vi "copy node from reference.vi"(8 "error in":errorcluster, 11 "TBM node dvr":refnum<data-value>) -> (0 "error out":errorcluster, 3 "TBM node value":refnum<class "TBM Configuration Node.lvclass">)   [LabVIEW 2013, in "PL Framework Configuration Tool.lvlib" / "TBM Configuration Node.lvclass"]
uses:
  TBM Configuration Node.lvclass
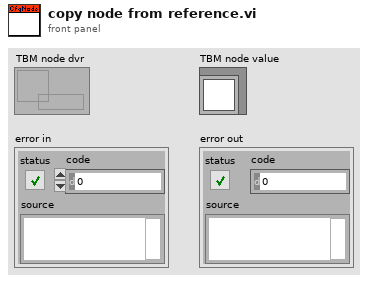
[diagram p1: front panel]
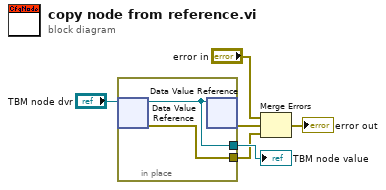
[diagram p0: block diagram]
diagram:
  n1 = in-place {
    in-place-border: [w8] -> w3
    in-place-border: [w7] -> w4
    n2 = in-place-dvr #1("TBM node dvr") -> (w7:refnum<class "TBM Configuration Node.lvclass">, w8:errorcluster)
    n3 = in-place-dvr #1(w7) -> (w2:errorcluster)  [unwired: 1 out]
  }
  "TBM node value" <- w4
  n4 = Merge Errors("error in", w2, w3) -> (→"error out":errorcluster)
